vi "OBD_init.vi"(8 "error in (no error)":errorcluster, 11 "VISA Refnum in":refnum<visa-resource-name>) -> (0 "error out":errorcluster, 3 "VISA Refnum out":refnum<visa-resource-name>)   [LabVIEW 2020]
panel:
  in  "0100":bool
  out "read 6":string
  in  "ATST64":bool
  out "read 5":string
  in  "ATS0":bool
  out "read 4":string
  in  "ATE0":bool
  out "read 3":string
  out "read 2":string
  in  "ATD":bool
  out "read":string
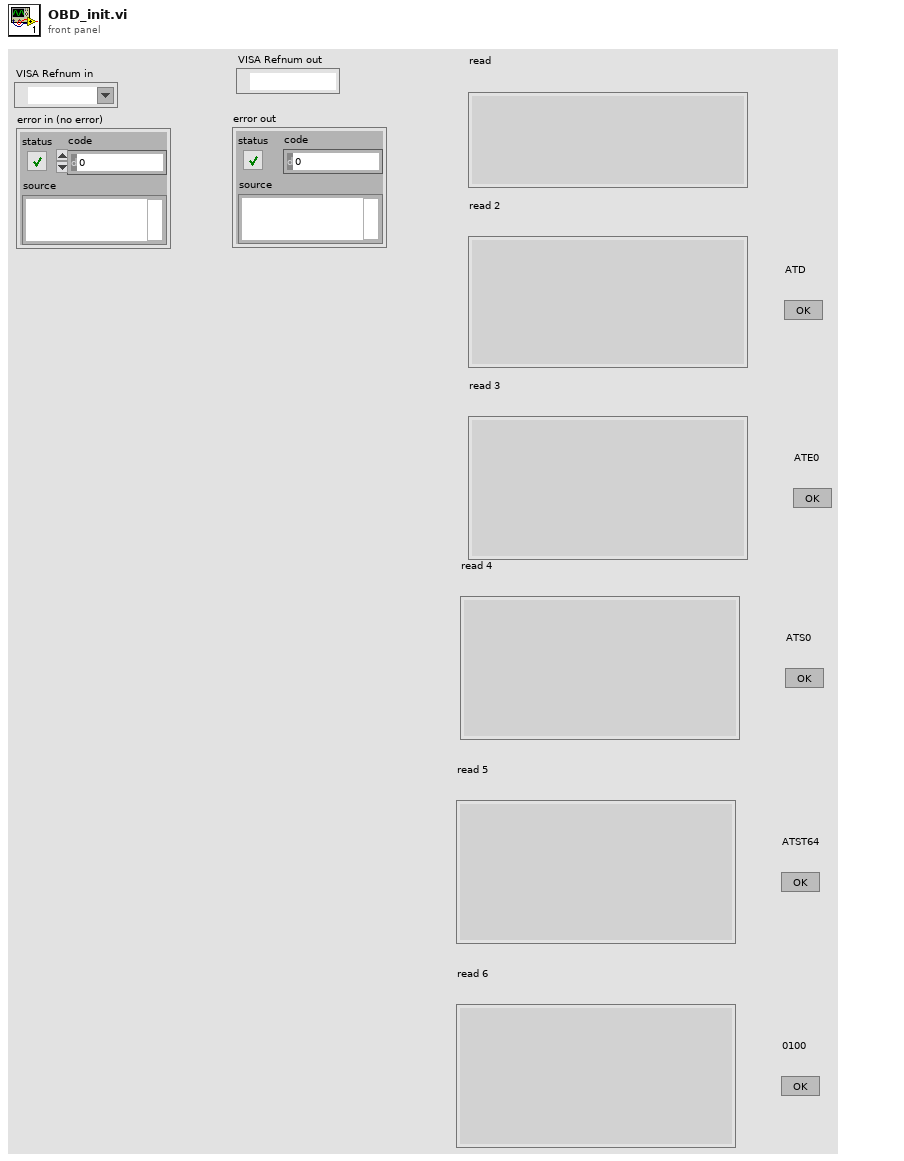
[diagram p1: front panel]
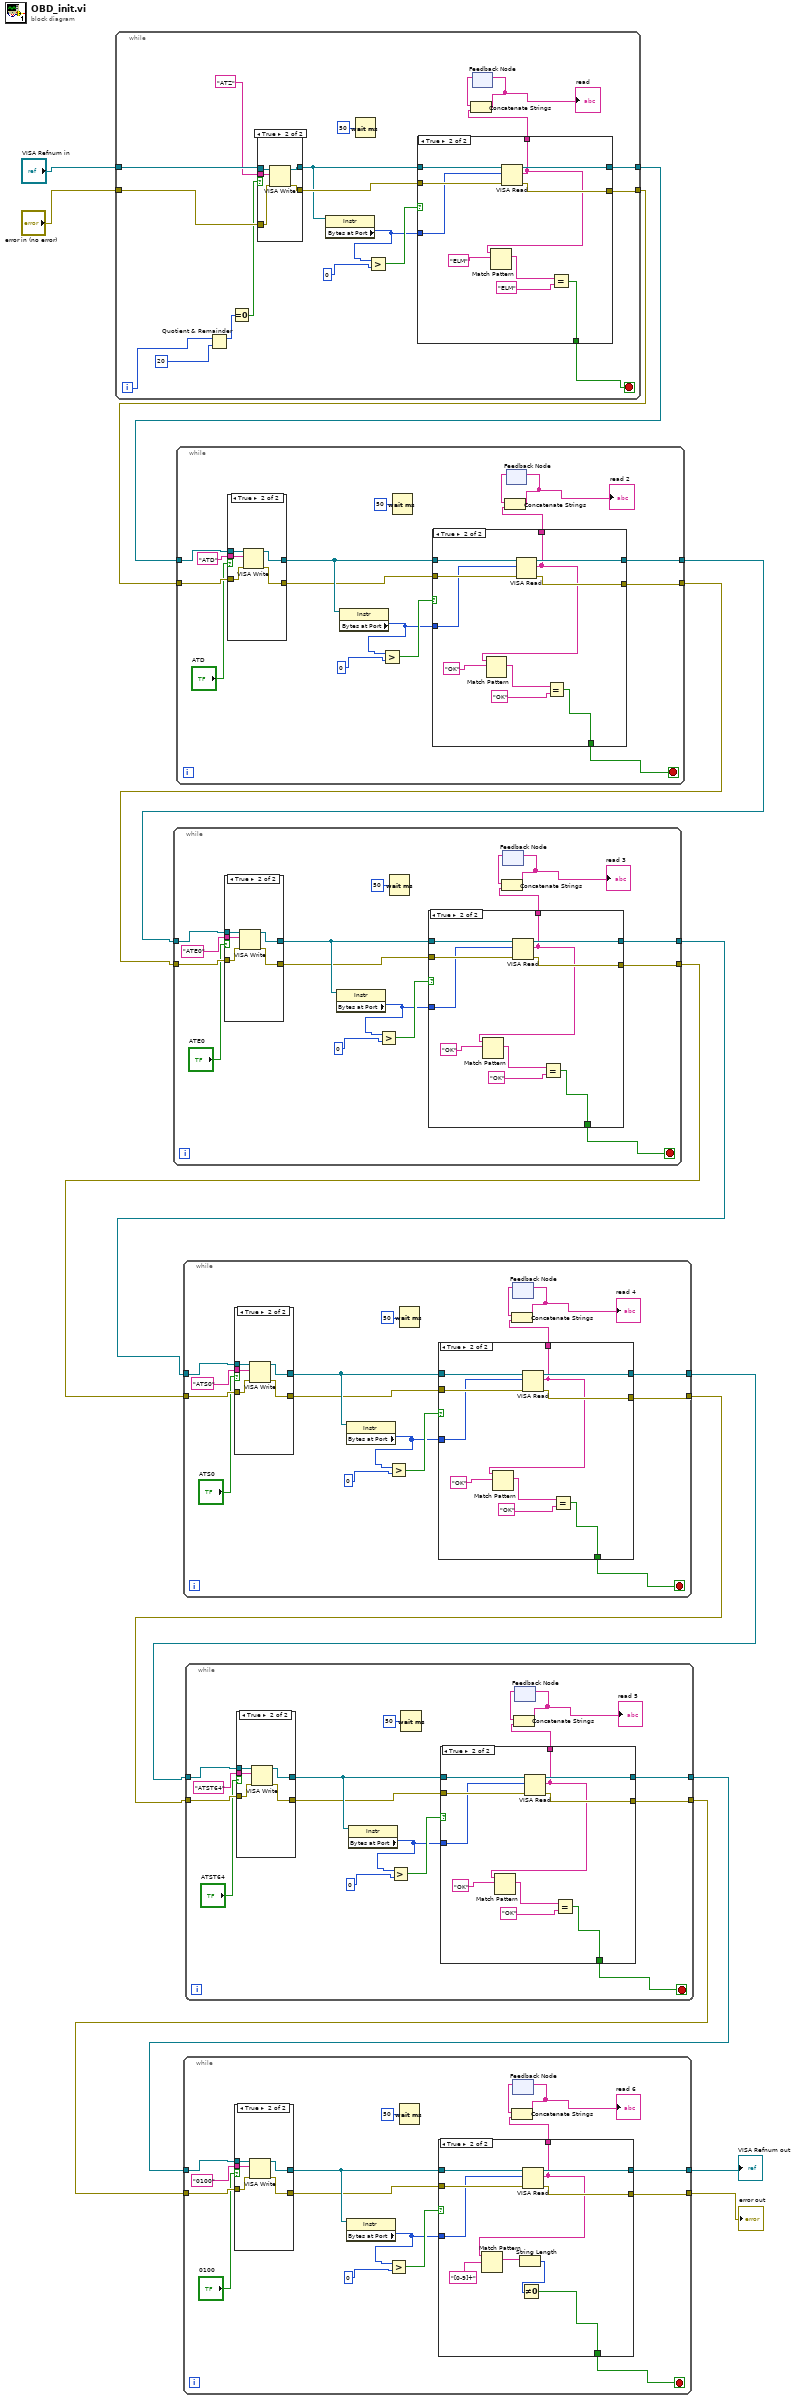
[diagram p0: block diagram]
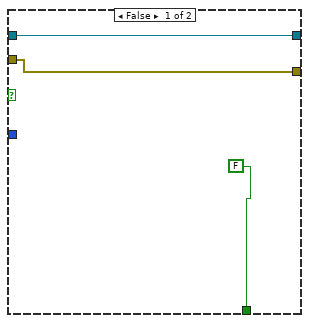
[diagram p3: hidden frame]
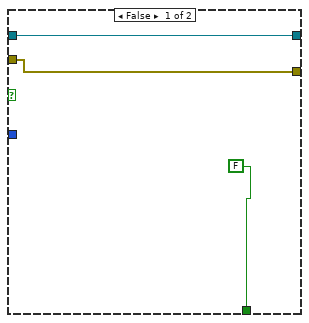
[diagram p5: hidden frame]
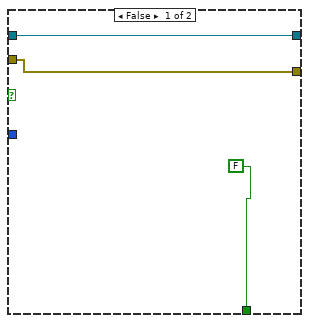
[diagram p7: hidden frame]
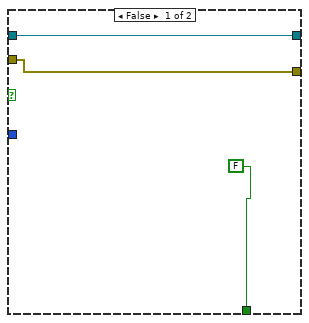
[diagram p9: hidden frame]
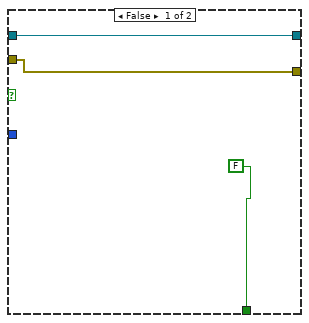
[diagram p11: hidden frame]
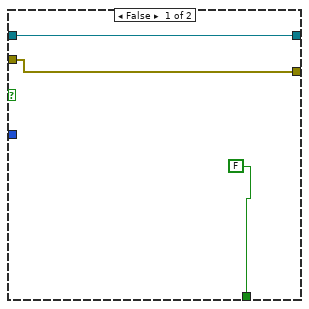
[diagram p13: hidden frame]
diagram:
  n1 = while {
    tunnel: "error in (no error)" -> [w32]
    tunnel: [w27] -> w11
    tunnel: "VISA Refnum in" -> [w33]
    tunnel: [w28] -> w12
    i -> [w15]
    stop <- w22 stop-if-true
    n2 = Quotient & Remainder(x=w15, y=20) -> (x-y*floor(x/y)=w17:i32)  [unwired: 1 out]
    n3 = Equal To 0?(x=w17) -> (x = 0?=w16:bool)
    n4 = case shown="True" w16 {
      tunnel: w33 -> [w35 w40]
      tunnel: w32 -> [w34 w39]
      tunnel: "ATZ" -> [_ w38]
      tunnel: [w34 w37] -> w30
      tunnel: [w35 w36] -> w29
      frame False {
      }
      frame True {
        n5 = VISA Write(VISA resource name=w40, write buffer=w38, error in (no error)=w39) -> (VISA resource name out=w36:refnum<visa-resource-name>, error out=w37:errorcluster)  [unwired: 1 out]
      }
    }
    n6 = property class="Instr"(reference=w29) -> ("Bytes at Port"=w25:u32)  [unwired: 1 in, 2 out]
    n7 = Wait (ms)(milliseconds to wait=u32 50) -> ()  [unwired: 1 out]
    n8 = Greater?(x=w25, y=u32 0) -> (0:w26:bool)
    n9 = case shown="True" w26 {
      tunnel: w30 -> [w43 w53]
      tunnel: w25 -> [_ w52]
      tunnel: w29 -> [w42 w51]
      tunnel: [w42 w50] -> w28
      tunnel: [w43 w49] -> w27
      tunnel: [FALSE w44] -> w22
      tunnel: [_ w45] -> w19
      frame False {
      }
      frame True {
        n10 = VISA Read(VISA resource name=w51, byte count=w52, error in (no error)=w53) -> (VISA resource name out=w50:refnum<visa-resource-name>, read buffer=w45:string, error out=w49:errorcluster)  [unwired: 1 out]
        n11 = Match Pattern(string=w45, regular expression="ELM") -> (match substring=w46:string)  [unwired: 1 in, 3 out]
        n12 = Equal?(x=w46, y="ELM") -> (x = y?=w44:bool)
      }
    }
    n13 = feedback #1() -> (w21:string)  [unwired: 1 in]
    n14 = Concatenate Strings(w21, w19) -> (w20:string)
    "read" <- w20
    n15 = feedback-in #1(w20) -> ()
  }
  n16 = while {
    tunnel: w12 -> [w68]
    tunnel: [w64] -> w10
    tunnel: w11 -> [w67]
    tunnel: [w63] -> w9
    stop <- w58 stop-if-true
    n17 = case shown="True" "ATD" {
      tunnel: "ATD" -> [_ w76]
      tunnel: w68 -> [w71 w75]
      tunnel: w67 -> [w70 w74]
      tunnel: [w71 w73] -> w66
      tunnel: [w70 w72] -> w65
      frame False {
      }
      frame True {
        n18 = VISA Write(VISA resource name=w75, write buffer=w76, error in (no error)=w74) -> (VISA resource name out=w73:refnum<visa-resource-name>, error out=w72:errorcluster)  [unwired: 1 out]
      }
    }
    n19 = property class="Instr"(reference=w66) -> ("Bytes at Port"=w61:u32)  [unwired: 1 in, 2 out]
    n20 = Greater?(x=w61, y=u32 0) -> (0:w62:bool)
    n21 = Wait (ms)(milliseconds to wait=u32 50) -> ()  [unwired: 1 out]
    n22 = case shown="True" w62 {
      tunnel: w65 -> [w79 w89]
      tunnel: w61 -> [_ w88]
      tunnel: w66 -> [w78 w87]
      tunnel: [w78 w86] -> w64
      tunnel: [w79 w85] -> w63
      tunnel: [FALSE w82] -> w58
      tunnel: [_ w83] -> w54
      frame False {
      }
      frame True {
        n23 = VISA Read(VISA resource name=w87, byte count=w88, error in (no error)=w89) -> (VISA resource name out=w86:refnum<visa-resource-name>, read buffer=w83:string, error out=w85:errorcluster)  [unwired: 1 out]
        n24 = Match Pattern(string=w83, regular expression="OK") -> (match substring=w80:string)  [unwired: 1 in, 3 out]
        n25 = Equal?(x=w80, y="OK") -> (x = y?=w82:bool)
      }
    }
    n26 = feedback #2() -> (w56:string)  [unwired: 1 in]
    n27 = Concatenate Strings(w56, w54) -> (w55:string)
    "read 2" <- w55
    n28 = feedback-in #2(w55) -> ()
  }
  n29 = while {
    tunnel: w10 -> [w104]
    tunnel: [w100] -> w7
    tunnel: w9 -> [w103]
    tunnel: [w99] -> w8
    stop <- w94 stop-if-true
    n30 = case shown="True" "ATE0" {
      tunnel: "ATE0" -> [_ w112]
      tunnel: w104 -> [w107 w111]
      tunnel: w103 -> [w106 w110]
      tunnel: [w107 w109] -> w102
      tunnel: [w106 w108] -> w101
      frame False {
      }
      frame True {
        n31 = VISA Write(VISA resource name=w111, write buffer=w112, error in (no error)=w110) -> (VISA resource name out=w109:refnum<visa-resource-name>, error out=w108:errorcluster)  [unwired: 1 out]
      }
    }
    n32 = property class="Instr"(reference=w102) -> ("Bytes at Port"=w97:u32)  [unwired: 1 in, 2 out]
    n33 = Greater?(x=w97, y=u32 0) -> (0:w98:bool)
    n34 = Wait (ms)(milliseconds to wait=u32 50) -> ()  [unwired: 1 out]
    n35 = case shown="True" w98 {
      tunnel: w101 -> [w115 w125]
      tunnel: w97 -> [_ w124]
      tunnel: w102 -> [w114 w123]
      tunnel: [w114 w122] -> w100
      tunnel: [w115 w121] -> w99
      tunnel: [FALSE w118] -> w94
      tunnel: [_ w119] -> w90
      frame False {
      }
      frame True {
        n36 = VISA Read(VISA resource name=w123, byte count=w124, error in (no error)=w125) -> (VISA resource name out=w122:refnum<visa-resource-name>, read buffer=w119:string, error out=w121:errorcluster)  [unwired: 1 out]
        n37 = Match Pattern(string=w119, regular expression="OK") -> (match substring=w116:string)  [unwired: 1 in, 3 out]
        n38 = Equal?(x=w116, y="OK") -> (x = y?=w118:bool)
      }
    }
    n39 = feedback #3() -> (w92:string)  [unwired: 1 in]
    n40 = Concatenate Strings(w92, w90) -> (w91:string)
    "read 3" <- w91
    n41 = feedback-in #3(w91) -> ()
  }
  n42 = while {
    tunnel: w7 -> [w140]
    tunnel: [w136] -> w6
    tunnel: w8 -> [w139]
    tunnel: [w135] -> w5
    stop <- w130 stop-if-true
    n43 = case shown="True" "ATS0" {
      tunnel: "ATS0" -> [_ w148]
      tunnel: w140 -> [w143 w147]
      tunnel: w139 -> [w142 w146]
      tunnel: [w143 w145] -> w138
      tunnel: [w142 w144] -> w137
      frame False {
      }
      frame True {
        n44 = VISA Write(VISA resource name=w147, write buffer=w148, error in (no error)=w146) -> (VISA resource name out=w145:refnum<visa-resource-name>, error out=w144:errorcluster)  [unwired: 1 out]
      }
    }
    n45 = property class="Instr"(reference=w138) -> ("Bytes at Port"=w133:u32)  [unwired: 1 in, 2 out]
    n46 = Greater?(x=w133, y=u32 0) -> (0:w134:bool)
    n47 = Wait (ms)(milliseconds to wait=u32 50) -> ()  [unwired: 1 out]
    n48 = case shown="True" w134 {
      tunnel: w137 -> [w151 w161]
      tunnel: w133 -> [_ w160]
      tunnel: w138 -> [w150 w159]
      tunnel: [w150 w158] -> w136
      tunnel: [w151 w157] -> w135
      tunnel: [FALSE w154] -> w130
      tunnel: [_ w155] -> w126
      frame False {
      }
      frame True {
        n49 = VISA Read(VISA resource name=w159, byte count=w160, error in (no error)=w161) -> (VISA resource name out=w158:refnum<visa-resource-name>, read buffer=w155:string, error out=w157:errorcluster)  [unwired: 1 out]
        n50 = Match Pattern(string=w155, regular expression="OK") -> (match substring=w152:string)  [unwired: 1 in, 3 out]
        n51 = Equal?(x=w152, y="OK") -> (x = y?=w154:bool)
      }
    }
    n52 = feedback #4() -> (w128:string)  [unwired: 1 in]
    n53 = Concatenate Strings(w128, w126) -> (w127:string)
    "read 4" <- w127
    n54 = feedback-in #4(w127) -> ()
  }
  n55 = while {
    tunnel: w6 -> [w176]
    tunnel: [w172] -> w3
    tunnel: w5 -> [w175]
    tunnel: [w171] -> w4
    stop <- w166 stop-if-true
    n56 = case shown="True" "ATST64" {
      tunnel: "ATST64" -> [_ w184]
      tunnel: w176 -> [w179 w183]
      tunnel: w175 -> [w178 w182]
      tunnel: [w179 w181] -> w174
      tunnel: [w178 w180] -> w173
      frame False {
      }
      frame True {
        n57 = VISA Write(VISA resource name=w183, write buffer=w184, error in (no error)=w182) -> (VISA resource name out=w181:refnum<visa-resource-name>, error out=w180:errorcluster)  [unwired: 1 out]
      }
    }
    n58 = property class="Instr"(reference=w174) -> ("Bytes at Port"=w169:u32)  [unwired: 1 in, 2 out]
    n59 = Greater?(x=w169, y=u32 0) -> (0:w170:bool)
    n60 = Wait (ms)(milliseconds to wait=u32 50) -> ()  [unwired: 1 out]
    n61 = case shown="True" w170 {
      tunnel: w173 -> [w187 w197]
      tunnel: w169 -> [_ w196]
      tunnel: w174 -> [w186 w195]
      tunnel: [w186 w194] -> w172
      tunnel: [w187 w193] -> w171
      tunnel: [FALSE w190] -> w166
      tunnel: [_ w191] -> w162
      frame False {
      }
      frame True {
        n62 = VISA Read(VISA resource name=w195, byte count=w196, error in (no error)=w197) -> (VISA resource name out=w194:refnum<visa-resource-name>, read buffer=w191:string, error out=w193:errorcluster)  [unwired: 1 out]
        n63 = Match Pattern(string=w191, regular expression="OK") -> (match substring=w188:string)  [unwired: 1 in, 3 out]
        n64 = Equal?(x=w188, y="OK") -> (x = y?=w190:bool)
      }
    }
    n65 = feedback #5() -> (w164:string)  [unwired: 1 in]
    n66 = Concatenate Strings(w164, w162) -> (w163:string)
    "read 5" <- w163
    n67 = feedback-in #5(w163) -> ()
  }
  n68 = while {
    tunnel: w3 -> [w212]
    tunnel: [w208] -> w2
    tunnel: w4 -> [w211]
    tunnel: [w207] -> w1
    stop <- w202 stop-if-true
    n69 = case shown="True" "0100" {
      tunnel: "0100" -> [_ w220]
      tunnel: w212 -> [w215 w219]
      tunnel: w211 -> [w214 w218]
      tunnel: [w215 w217] -> w210
      tunnel: [w214 w216] -> w209
      frame False {
      }
      frame True {
        n70 = VISA Write(VISA resource name=w219, write buffer=w220, error in (no error)=w218) -> (VISA resource name out=w217:refnum<visa-resource-name>, error out=w216:errorcluster)  [unwired: 1 out]
      }
    }
    n71 = property class="Instr"(reference=w210) -> ("Bytes at Port"=w205:u32)  [unwired: 1 in, 2 out]
    n72 = Greater?(x=w205, y=u32 0) -> (0:w206:bool)
    n73 = Wait (ms)(milliseconds to wait=u32 50) -> ()  [unwired: 1 out]
    n74 = case shown="True" w206 {
      tunnel: w209 -> [w223 w233]
      tunnel: w205 -> [_ w232]
      tunnel: w210 -> [w222 w231]
      tunnel: [w222 w230] -> w208
      tunnel: [w223 w229] -> w207
      tunnel: [FALSE w226] -> w202
      tunnel: [_ w225] -> w198
      frame False {
      }
      frame True {
        n75 = VISA Read(VISA resource name=w231, byte count=w232, error in (no error)=w233) -> (VISA resource name out=w230:refnum<visa-resource-name>, read buffer=w225:string, error out=w229:errorcluster)  [unwired: 1 out]
        n76 = Match Pattern(string=w225, regular expression="[0-9]+") -> (match substring=w227:string)  [unwired: 1 in, 3 out]
        n77 = String Length(string=w227) -> (length=w224:i32)
        n78 = Not Equal To 0?(x=w224) -> (x != 0?=w226:bool)
      }
    }
    n79 = feedback #6() -> (w200:string)  [unwired: 1 in]
    n80 = Concatenate Strings(w200, w198) -> (w199:string)
    "read 6" <- w199
    n81 = feedback-in #6(w199) -> ()
  }
  "VISA Refnum out" <- w2
  "error out" <- w1
